vi "Open Device (index).vi"(8 "error in (no error)":errorcluster, 10 "Device Index":i32) -> (0 "error out":errorcluster, 3 "Handle":u64)   [LabVIEW 2019, in "D2XX-lv.lvlib"]
doc: "Open the specified device and return a handle that will be used for subsequent accesses. The device is specified by its index."
uses:
  D2XX-lv.lvlib
  <instrlib>/_D2XX/D2XX/D2XX.lvlib
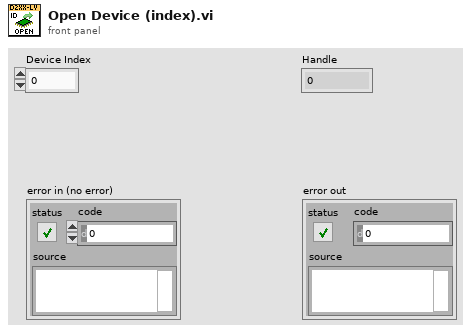
[diagram p1: front panel]
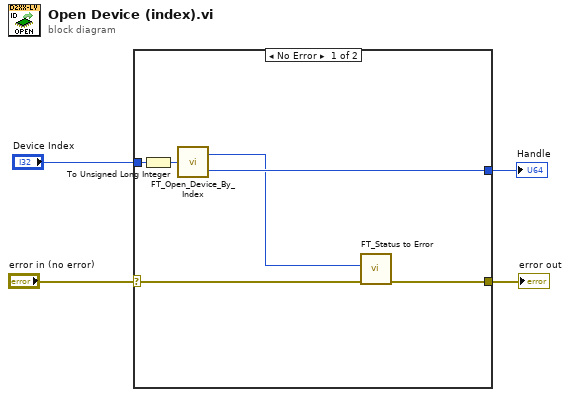
[diagram p0: block diagram]
diagram:
  n1 = case shown="No Error" "error in (no error)" {
    selector: "error in (no error)" -> [w10 w11]
    tunnel: [w9 w11] -> w3
    tunnel: "Device Index" -> [w8 _]
    tunnel: [w7 _] -> w1
    frame No Error {
      n2 = To Unsigned Long Integer(number=w8) -> (unsigned 32bit integer=w5:u32)
      n3 = call <instrlib>:"FT_Open_Device_By_Index.vi"("Device Index"=w5) -> ("FT_Status"=w6:u32, "Handle"=w7:u64)
      n4 = call "FT_Status to Error.vi"("error in (no error)"=w10, "FT_Status"=w6) -> ("error out"=w9:errorcluster)  [unwired: 9 in]
    }
    frame Error {
    }
  }
  "error out" <- w3
  "Handle" <- w1
